vi "Encrypt & Dycrypt.vi"(7 "Enum":enum16{"Encrypt", "Decrypt"}(ring), 8 "error in (no error)":errorcluster, 11 "Input":string) -> (0 "error out":errorcluster, 3 "Output":string)   [LabVIEW 2025]
panel:
  # "09_05_2026 USER SOFTWARE OPENED"
  # "`xdgr\trtdewl\nwt"
  # "1234567890 qwertyuiopasdfghjklzxcvbnm QWERTYUIOPASDFGHJKLZXCVBNM"
  # "as`gyw\n\t!6)&&65[_BW#%*3:%+^JJU&#\"9rwbfotwz|\n|}"
  # "6/19/2026-9:36 AM--------Platform Settings Button Pressed"
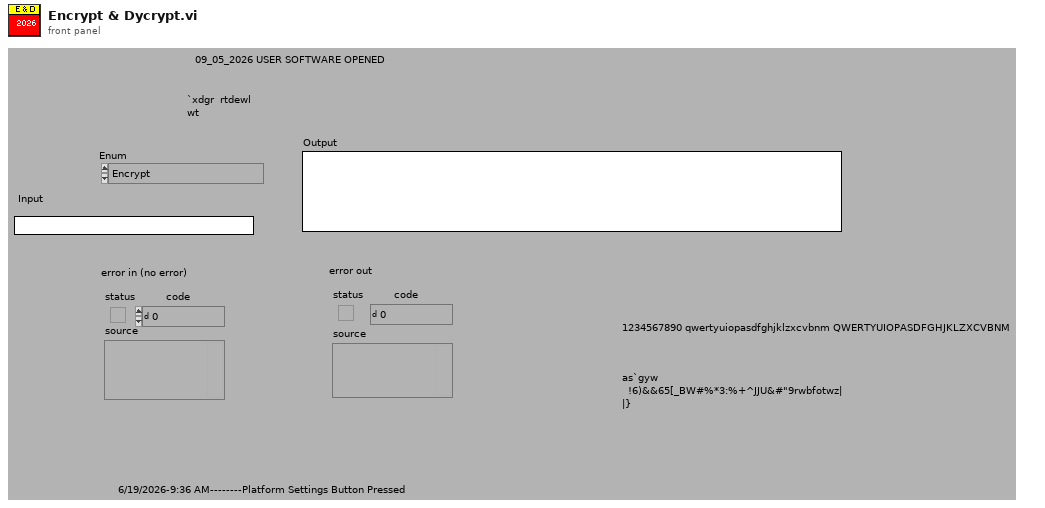
[diagram p1: front panel]
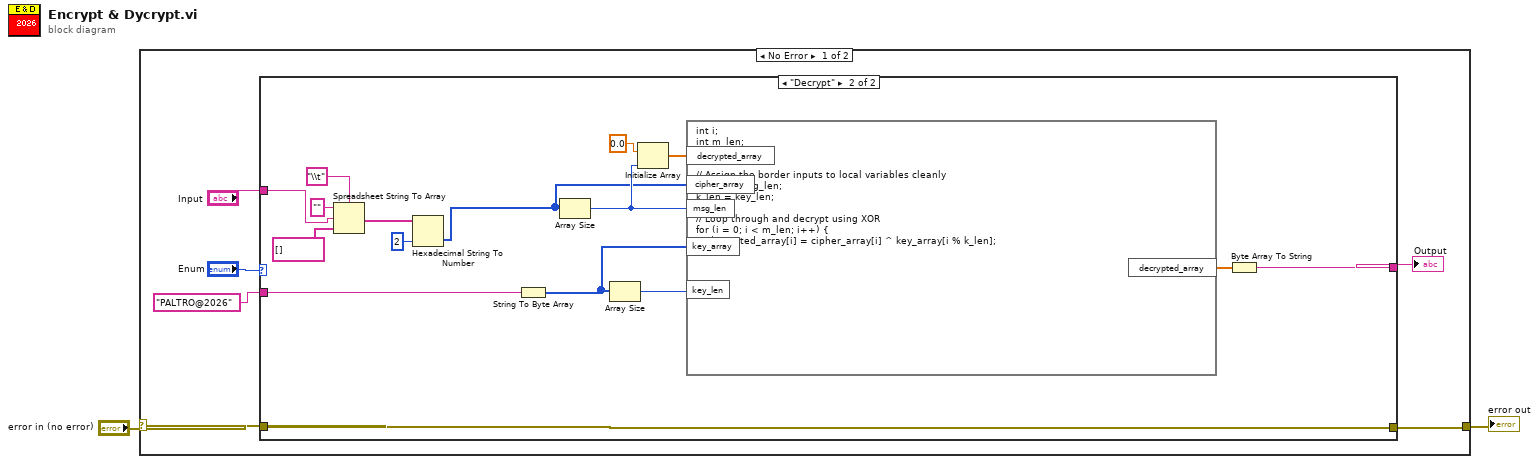
[diagram p0: block diagram]
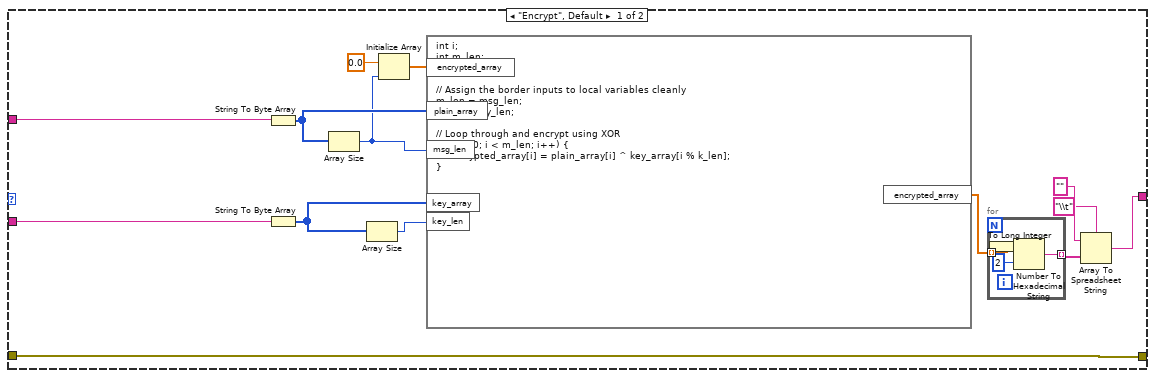
[diagram p2: hidden frame]
diagram:
  n1 = case shown="No Error" "error in (no error)" {
    selector: "error in (no error)" -> [w7 _]
    tunnel: [w5 _] -> w1
    frame No Error {
      n2 = case shown="\"Decrypt\"" "Enum" {
        tunnel: w7 -> [w22 w42]
        tunnel: "Input" -> [w21 w33]
        tunnel: [w22 w42] -> w5
        tunnel: "PALTRO@2026" -> [w19 w41]
        tunnel: [w10 w34] -> w3
        frame "Encrypt", Default {
          n3 = String To Byte Array(string=w21) -> (unsigned byte array=w20:u8[])
          n4 = String To Byte Array(string=w19) -> (unsigned byte array=w17:u8[])
          n5 = Array Size(array=w20) -> (size(s)=w15:i32)
          n6 = Array Size(array=w17) -> (size(s)=w18:i32)
          n7 = Initialize Array(0.0 ("element"), w15) -> (w14:dbl[])
          n8 = formula code="int i;\nint m_len;\nint k_len;\n\n// Assign the border inputs to local variables cleanly\nm_len = msg_len;\nk_len = key_len;\n\n// Loop through and encrypt using XOR\nfor (i = 0; i < m_len; i++) {\n    encrypted_array[i] = plain_array[i] ^ key_array[i % k_len];\n}"("plain_array"=w20, "key_array"=w17, "msg_len"=w15, "key_len"=w18, "encrypted_array"=w14) -> ("encrypted_array"=w13:dbl[])
          n9 = for {
            tunnel: w13 -> [w26] mode=indexing
            tunnel: [w25] -> w12 mode=indexing
            n10 = To Long Integer(number=w26) -> (32bit integer=w23:i32)
            n11 = Number To Hexadecimal String(1:i16 2 ("width (-)"), 2:w23) -> (0:w25:string)
          }
          n12 = Array To Spreadsheet String(delimiter (Tab)="\\t", array=w12, 3:"" ("format string")) -> (spreadsheet string=w10:string)
        }
        frame "Decrypt" {
          n13 = Spreadsheet String To Array(delimiter (Tab)="\\t", format string="", spreadsheet string=w33, array type (2D Dbl)=string[] []) -> (array=w29:string[])
          n14 = Hexadecimal String To Number(string=w29, default (0uL)=u32 2 ("default (0 U32)")) -> (number=w28:u32[])  [unwired: 1 in, 1 out]
          n15 = String To Byte Array(string=w41) -> (unsigned byte array=w40:u8[])
          n16 = Array Size(array=w28) -> (size(s)=w37:i32)
          n17 = Array Size(array=w40) -> (size(s)=w39:i32)
          n18 = Initialize Array(0.0 ("element"), w37) -> (w36:dbl[])
          n19 = formula code="int i;\nint m_len;\nint k_len;\n\n// Assign the border inputs to local variables cleanly\nm_len = msg_len;\nk_len = key_len;\n\n// Loop through and decrypt using XOR\nfor (i = 0; i < m_len; i++) {\n    decrypted_array[i] = cipher_array[i] ^ key_array[i % k_len];\n}"("cipher_array"=w28, "key_array"=w40, "msg_len"=w37, "key_len"=w39, "decrypted_array"=w36) -> ("decrypted_array"=w35:dbl[])
          n20 = Byte Array To String(unsigned byte array=w35) -> (string=w34:string)
        }
      }
      "Output" <- w3
    }
    frame Error {
    }
  }
  "error out" <- w1
